vi "ConfigAcq.vi"(8 "error in (no error)":errorcluster, 11 "DigitizerBase in":refnum<class "DigitizerBase.lvclass">) -> (0 "error out":errorcluster, 3 "DigitizerBase out":refnum<class "DigitizerBase.lvclass">)   [LabVIEW 2014, in "DigitizerPlugins.lvlib" / "DigitizerBase.lvclass"]
uses:
  DigitizerBase.lvclass
  DigitizerBase.lvclass/DigitizerBase.ctl
  Accessors/Read InstRef.vi
  Accessors/Read Acquisition.vi
  Accessors/Write InstRef.vi
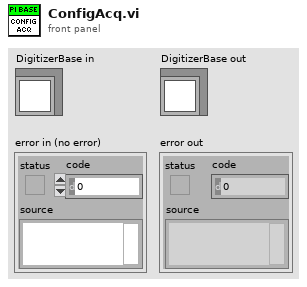
[diagram p1: front panel]
types:
  T1 = typedef "DigitizerPlugins.lvlib/DigitizerBase.lvclass/Acquisition.ctl" = cluster{"SampleRate":dbl, "RecordSize":i32, "NumRecords":i32, "SampleMode":i32, "Timeout (ms)":i32}
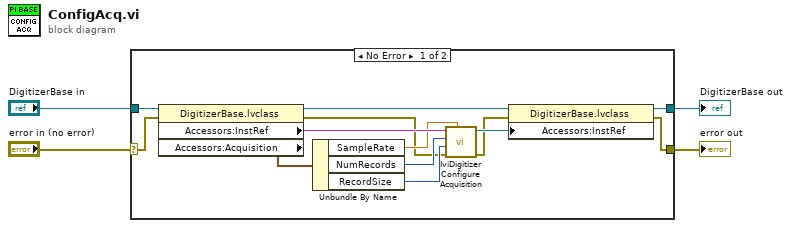
[diagram p0: block diagram]
diagram:
  n1 = case shown="No Error" "error in (no error)" {
    selector: "error in (no error)" -> [w15 w19]
    tunnel: [w5 w19] -> w3
    tunnel: [w8 w18] -> w1
    tunnel: "DigitizerBase in" -> [w17 w18]
    frame No Error {
      n2 = property class="DigitizerBase.lvclass"(reference=w17, error in=w15) -> (reference out=w16:refnum<class "DigitizerBase.lvclass">, error out=w9:errorcluster, "Accessors:InstRef"=w14:string, "Accessors:Acquisition"=w13:T1)
      n3 = Unbundle By Name(w13) -> ("SampleRate"=w12:dbl, "NumRecords"=w11:i32, "RecordSize"=w10:i32)
      n4 = call <vilib>:"IviDigitizer Configure Acquisition.vi"("Sample Rate (1.0e5)"=w12, "error in (no error)"=w9, "Record Size (256)"=w10, "Number of Records (1)"=w11, "instrument handle"=w14) -> ("error out"=w6:errorcluster, "instrument handle out"=w7:refnum<k15>)  [unwired: 5 in]
      n5 = property class="DigitizerBase.lvclass"(reference=w16, error in=w6, "Accessors:InstRef"=w7) -> (reference out=w8:refnum<class "DigitizerBase.lvclass">, error out=w5:errorcluster)
    }
    frame Error {
    }
  }
  "error out" <- w3
  "DigitizerBase out" <- w1
